vi "List Section Elements.vi"(8 "error in (no error)":errorcluster, 10 "Qualified Name":string, 11 "Attribute.Config in":refnum<class "Attribute.Config.lvclass">) -> (0 "error out":errorcluster, 2 "Keys":string[](array[string]), 3 "Attribute.Config out":refnum<class "Attribute.Config.lvclass">)   [LabVIEW 2013, in "Attribute.Config.lvclass"]
uses:
  Attribute.Config.lvclass
  Attribute.Config.lvclass/Attribute.Config.ctl
  <vilib>/LabVIEW Open Source/Configuration Manager/Manager/ConfigManager.lvclass
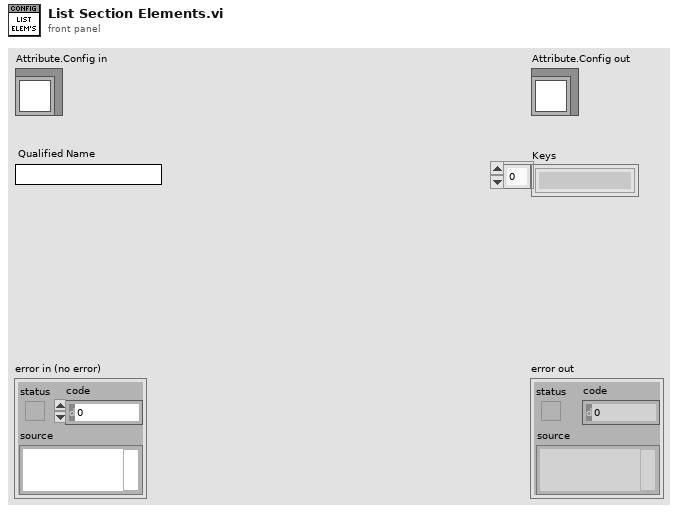
[diagram p1: front panel]
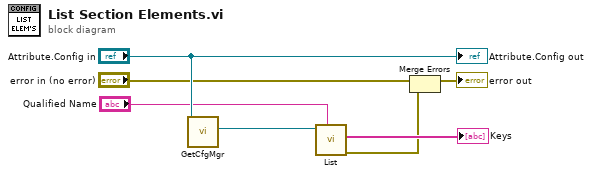
[diagram p0: block diagram]
diagram:
  n1 = call "GetCfgMgr.vi"("Attribute.Config in"="Attribute.Config in") -> ("CfgMgr"=w4:refnum<class "ConfigManager.lvclass">)  [unwired: 9 in, 1 out]
  n2 = call <vilib>:"List.vi"("Qualified Name"="Qualified Name", "ConfigManager in"=w4) -> ("error out"=w2:errorcluster, "Keys"=→"Keys":string[])  [unwired: 7 in, 1 out]
  n3 = Merge Errors("error in (no error)", w2) -> (→"error out":errorcluster)
  "Attribute.Config out" <- "Attribute.Config in"
